vi "ISO频率上下限.vi"(9 "麦克风间距s[mm]":dbl, 10 "管直径d[mm]":dbl, 11 "声速c":dbl) -> (2 "频率下限fL":dbl, 3 "频率上限fu":dbl)   [LabVIEW 2018]
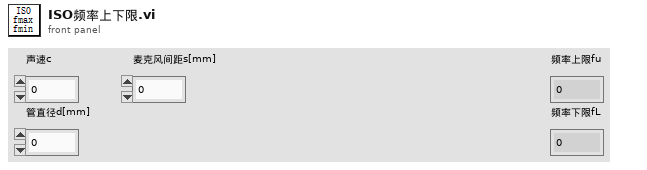
[diagram p1: front panel]
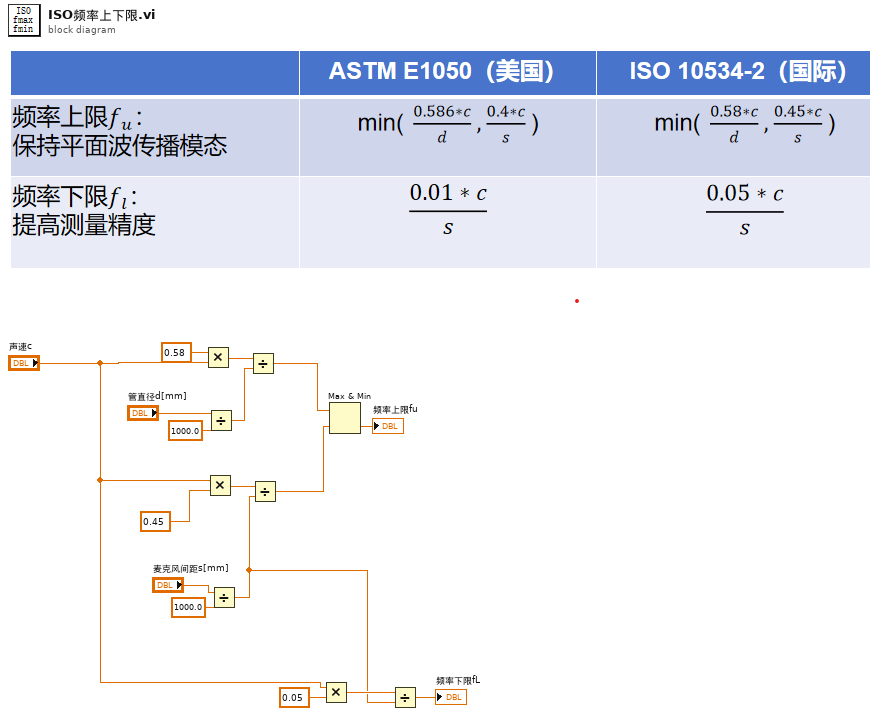
[diagram p0: block diagram]
diagram:
  n1 = Multiply(x=0.58, y="声速c") -> (x*y=w16:dbl)
  n2 = Multiply(x="声速c", y=0.45) -> (x*y=w14:dbl)
  n3 = Divide(x="管直径d[mm]", y=1000.0) -> (x/y=w11:dbl)
  n4 = Divide(x="麦克风间距s[mm]", y=1000.0) -> (x/y=w2:dbl)
  n5 = Divide(x=w16, y=w11) -> (x/y=w15:dbl)
  n6 = Divide(x=w14, y=w2) -> (x/y=w7:dbl)
  n7 = Multiply(x="声速c", y=0.05) -> (x*y=w3:dbl)
  n8 = Max & Min(x=w15, y=w7) -> (min(x,y)=→"频率上限fu":dbl)  [unwired: 1 out]
  n9 = Divide(x=w3, y=w2) -> (x/y=→"频率下限fL":dbl)
